vi "test_rigol_read.vi"() -> ()   [LabVIEW 2018]
panel:
  in  "VISA resource name":refnum<visa-resource-name>
  out "Waveform Graph":u8[](graph)
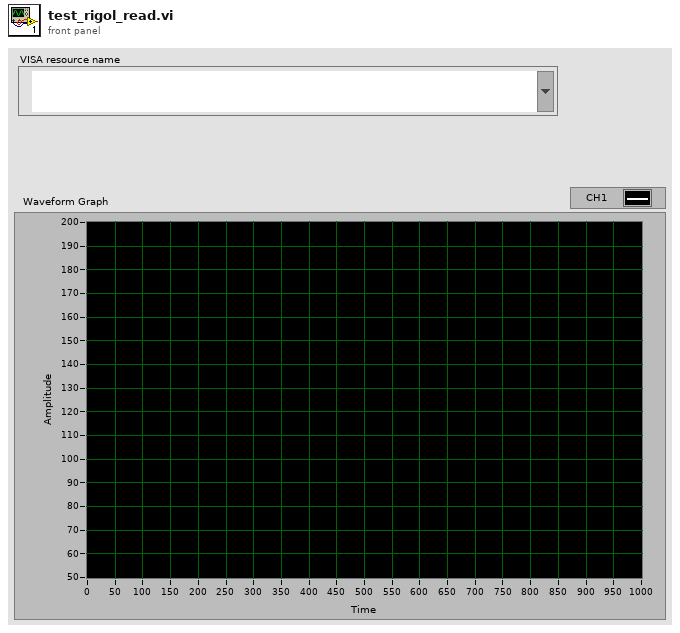
[diagram p1: front panel]
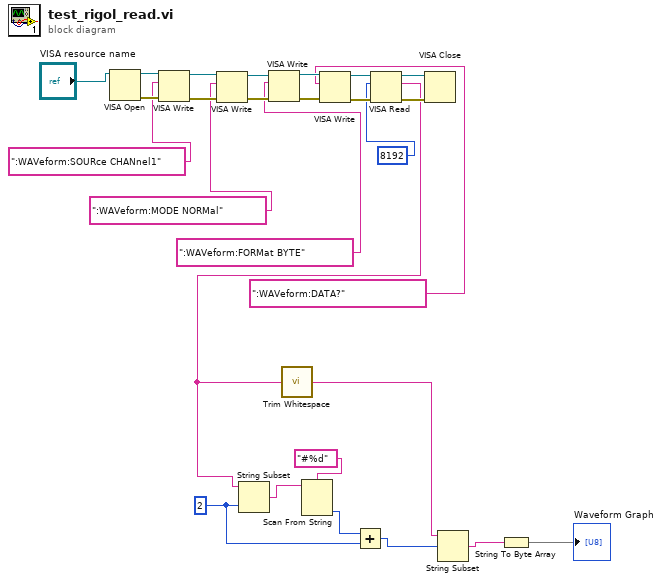
[diagram p0: block diagram]
diagram:
  w5 = 2
  n1 = VISA Open(VISA resource name="VISA resource name") -> (VISA resource name=w24:refnum<visa-resource-name>, error out=w23:errorcluster)  [unwired: 4 in]
  n2 = VISA Write(VISA resource name=w24, write buffer=":WAVeform:SOURce CHANnel1", error in (no error)=w23) -> (VISA resource name out=w21:refnum<visa-resource-name>, error out=w22:errorcluster)  [unwired: 1 out]
  n3 = VISA Write(VISA resource name=w21, write buffer=":WAVeform:MODE NORMal", error in (no error)=w22) -> (VISA resource name out=w20:refnum<visa-resource-name>, error out=w19:errorcluster)  [unwired: 1 out]
  n4 = VISA Write(VISA resource name=w20, write buffer=":WAVeform:FORMat BYTE", error in (no error)=w19) -> (VISA resource name out=w18:refnum<visa-resource-name>, error out=w17:errorcluster)  [unwired: 1 out]
  n5 = VISA Write(VISA resource name=w18, write buffer=":WAVeform:DATA?", error in (no error)=w17) -> (VISA resource name out=w16:refnum<visa-resource-name>, error out=w15:errorcluster)  [unwired: 1 out]
  n6 = VISA Read(VISA resource name=w16, byte count=8192, error in (no error)=w15) -> (VISA resource name out=w25:refnum<visa-resource-name>, read buffer=w7:string, error out=w26:errorcluster)  [unwired: 1 out]
  n7 = String Subset(string=w7, length (rest)=w5) -> (substring=w9:string)  [unwired: 1 in]
  n8 = call <vilib>:"Trim Whitespace.vi"("string"=w7) -> ("trimmed string"=w4:string)  [unwired: 1 in]
  n9 = Scan From String(format string="#%d", input string=w9) -> (output 1=w6:i32)  [unwired: 3 in, 3 out]
  n10 = Add(x=w6, y=w5) -> (x+y=w3:i32)
  n11 = VISA Close(VISA resource name=w25, error in (no error)=w26) -> ()  [unwired: 1 out]
  n12 = String Subset(string=w4, offset (0)=w3) -> (substring=w2:string)  [unwired: 1 in]
  n13 = String To Byte Array(string=w2) -> (unsigned byte array=→"Waveform Graph":u8[])
